vi "DAQ_make_global_channel.vi"(10 "DAQmx Physical Channel":tag) -> (2 "concatenated string":string)   [LabVIEW 2016]
uses:
  <vilib>/regexp/Match Regular Expression.xnode
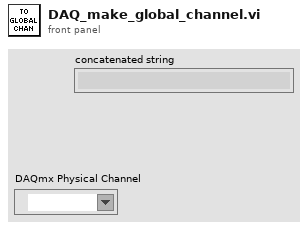
[diagram p1: front panel]
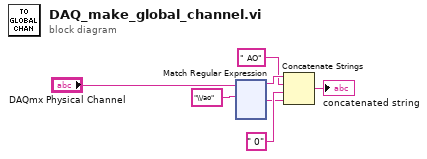
[diagram p0: block diagram]
diagram:
  n1 = xnode "Match Regular Expression"("input string"="DAQmx Physical Channel", "regular expression"="\\/ao") -> ("before match"=w5:string, "after match"=w2:string)  [unwired: 4 in, 3 out]
  n2 = Concatenate Strings(w5, " AO" ("string"), " 0" ("string"), w2) -> (→"concatenated string":string)
